vi "Clone.vi"(8 "error in (no error)":errorcluster, 11 "Object (subject) in":refnum<class "Object (subject).lvclass">) -> (0 "error out":errorcluster, 2 "clone":refnum<class "Object (subject).lvclass">, 3 "Object (subject) out":refnum<class "Object (subject).lvclass">)   [LabVIEW 2014, in "Object (subject).lvclass"]
uses:
  Object (subject).lvclass
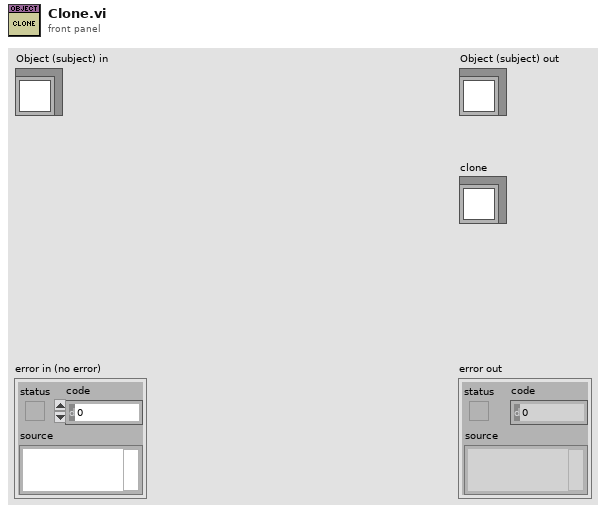
[diagram p1: front panel]
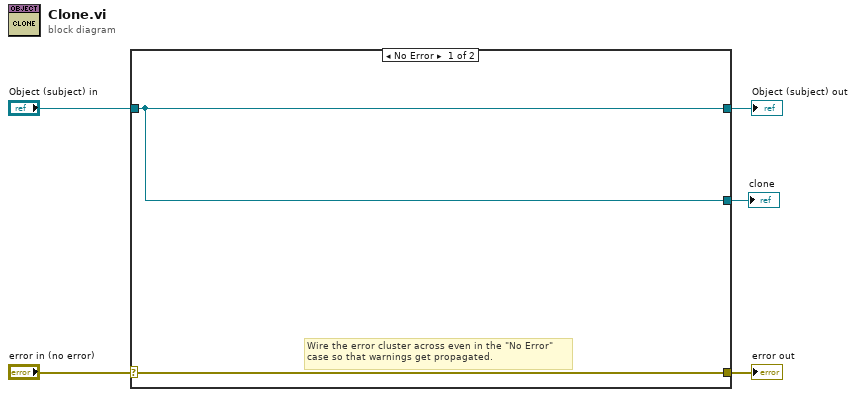
[diagram p0: block diagram]
diagram:
  n1 = case shown="No Error" "error in (no error)" {
    selector: "error in (no error)" -> [w7 w9]
    tunnel: [w7 w9] -> w4
    tunnel: [w6 w8] -> w2
    tunnel: "Object (subject) in" -> [w6 w8]
    tunnel: [w6 _] -> w1
    frame No Error {
      # "Wire the error cluster across even in the \"No Error\"\ncase so that warnings get propagated."
    }
    frame Error {
    }
  }
  "error out" <- w4
  "Object (subject) out" <- w2
  "clone" <- w1
